vi "Vagus Controller FUZZY ECG Continuous Keithley.vi"() -> ()   [LabVIEW 2020]
uses:
  <instrlib>/Keithley 622x LV 2009/Utility/Typedefs/KE622x -- Instrument Type.ctl
  <instrlib>/Keithley 622x LV 2009/Typedefs/KE622x -- On Off Control.ctl
  <instrlib>/Keithley 622x LV 2009/Configure/Output/Typedefs/KE6221 -- Output Response.ctl
  <instrlib>/Keithley 622x LV 2009/Configure/Source/Typedefs/KE622x -- Current Range.ctl
  <instrlib>/Keithley 622x LV 2009/Configure/Source/Typedefs/KE622x -- Current Ranges.ctl
  <instrlib>/Keithley 622x LV 2009/Configure/Source/Typedefs/KE622x -- Voltage Limit.ctl
  <instrlib>/Keithley 622x LV 2009/Utility/Typedefs/KE622x -- Serial Port Settings.ctl
  <instrlib>/Keithley 622x LV 2009/Configure/Source/Typedefs/KE622x -- Current Level.ctl
  <vilib>/Analysis/baseanly.llb/Mean (DBL).vi
  <vilib>/measure/mascope.llb/Pulse Measurements 1 chan.vi
  <vilib>/addons/Fuzzy Logic/FL Fuzzy Controller (MISO).vi
  <vilib>/Utility/file.llb/Write Delimited Spreadsheet (DBL).vi
  <vilib>/measure/NI_MAPro.lvlib
  <vilib>/addons/Fuzzy Logic/NI_Fuzzy_Logic_API.lvlib
  <instrlib>/Keithley 622x LV 2009/Keithley 622x.lvlib
  <vilib>/Analysis/NI_AALBase.lvlib
panel:
  out "Charge\nDelivered (mC)":dbl
  in  "Reset Charge":bool
  in  "Num Samples\nHR Median":i64 max=1000
  in  "Num Samples\nDC Remove":i64 max=1000
  in  "File Name":string
  in  "Pulse \nPolarity":u16(ring)=1 items=["low pulse", "high pulse"]
  out "Smoothed HR:":dbl format="%#_4g"
  out "Rules Used by Fuzzy Controller":cluster{"Color Box":u32, string}[](array[cluster])
  in  "Activate Controller":bool
  in  "Gain Multiplier":ext
  in  "HR Beat\nThreshold (V)":dbl
  out "?":bool
  out "Measured HR :":dbl format="%#_4g"
  out "HR Waveform":waveform(dbl)(graph)
  in  "Min Current (mA)":dbl
  in  "Max Current (mA)":dbl
  in  "Length of \nBuffer (s)":dbl
  out "Block Output (mA)":ext(graph)
  out "HR Chart":cluster{dbl, "HR Setpoint":i64}(graph)
  in  "HR Setpoint":i64(slide)=200 min=100 max=450 step=1 scale=175.0..375.0
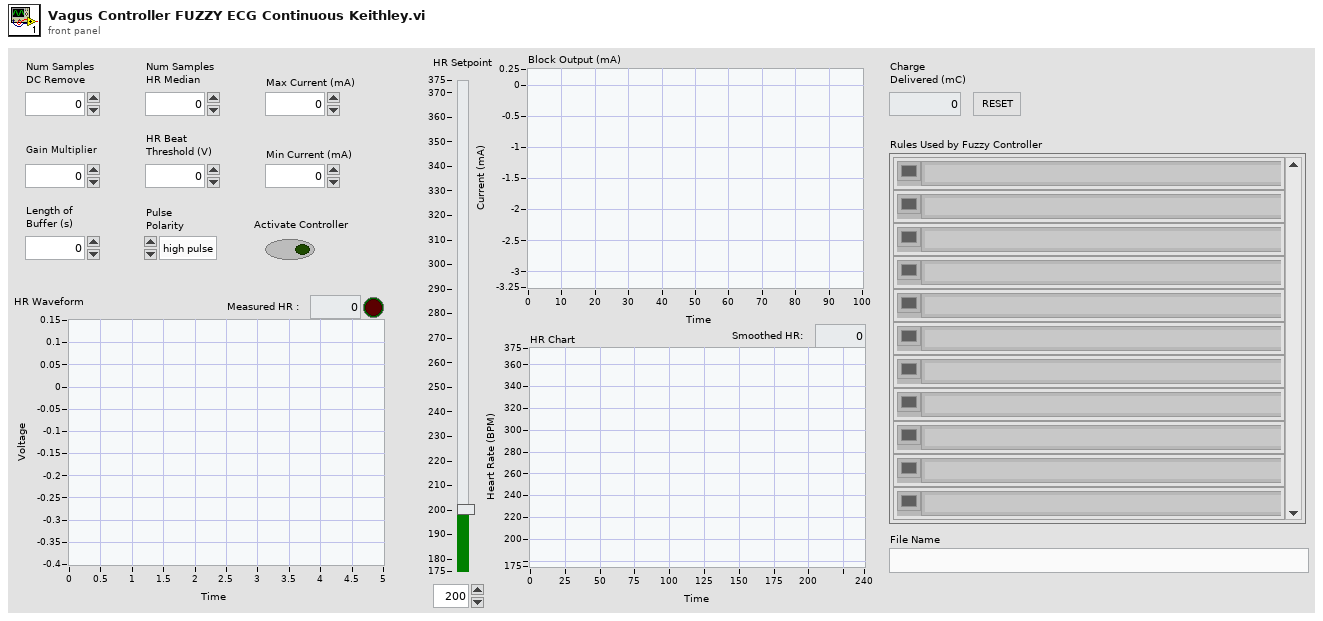
[diagram p1: front panel]
types:
  T1 = typedef "Keithley 622x.lvlib/KE622x -- Current Level.ctl" = dbl
  T2 = typedef "Keithley 622x.lvlib/KE622x -- On Off Control.ctl" = enum16{"Off", "On"}
  T3 = typedef "Keithley 622x.lvlib/KE622x -- Serial Port Settings.ctl" = cluster{"Read Term Char":enum16{"CR", "LF", "CR + LF", "LF + CR"}, "Baud Rate":enum16{"300", "600", "1200", "2400", "4800", "9600", "19200", "38400", "57600", "115200"}, "Flow Control\n(XON / XOFF)":enum16{"Off", "On"}}
  T4 = typedef "Keithley 622x.lvlib/KE622x -- Voltage Limit.ctl" = dbl
  T5 = typedef "Keithley 622x.lvlib/KE622x -- Current Range.ctl" = cluster{"Auto Range?":bool, "Man / Selected\nRange":T6}
  T6 = typedef "Keithley 622x.lvlib/KE622x -- Current Ranges.ctl" = enum16{"2nA", "20nA", "200nA", "2uA", "20uA", "200uA", "2mA", "20mA", "100mA"}
  T7 = typedef "Keithley 622x.lvlib/KE6221 -- Output Response.ctl" = enum16{"Fast", "Slow"}
  T8 = typedef "Keithley 622x.lvlib/KE622x -- Instrument Type.ctl" = enum16{"KE6220", "KE6221"}
  T9 = enum16{"open", "replace", "create", "open or create", "replace or create", "replace or create with confirmation"}
  T10 = typedef "NI_Fuzzy_Logic_API.lvlib/FL System.ctl" = cluster{"input variables":T11[], "output variables":T11[], "rules":T14[], "defuzzification method":T20, "description":string, "user MF interpolating polynomials":T21[]}
  T11 = typedef "NI_Fuzzy_Logic_API.lvlib/FL Variable.ctl" = cluster{"name":string, "range":dbl[], "MFs":T12[]}
  T12 = typedef "NI_Fuzzy_Logic_API.lvlib/FL Membership Function.ctl" = cluster{"name":string, "shape":T13, "points":dbl[], "color":u32, "user-defined shape index":i32}
  T13 = typedef "NI_Fuzzy_Logic_API.lvlib/FL Membership Function Shape.ctl" = u16
  T14 = typedef "NI_Fuzzy_Logic_API.lvlib/FL Rule.ctl" = cluster{"antecedents":T15[], "antecedent connective":T17, "consequents":T18[], "consequent implication":T19, "degree of support":dbl}
  T15 = typedef "NI_Fuzzy_Logic_API.lvlib/FL Antecedent.ctl" = cluster{"Var Index":i32, "MF Index":i32, "Cond":T16}
  T16 = typedef "NI_Fuzzy_Logic_API.lvlib/FL Modifier.ctl" = u16
  T17 = typedef "NI_Fuzzy_Logic_API.lvlib/FL Antecedent Connective.ctl" = u16
  T18 = typedef "NI_Fuzzy_Logic_API.lvlib/FL Consequent.ctl" = cluster{"Var Index":i32, "MF Index":i32, "Cond":T16}
  T19 = typedef "NI_Fuzzy_Logic_API.lvlib/FL Consequent Implication.ctl" = u16
  T20 = typedef "NI_Fuzzy_Logic_API.lvlib/FL Defuzzification.ctl" = u16
  T21 = typedef "NI_Fuzzy_Logic_API.lvlib/FL Interpolating polynomials.ctl" = cluster{"X":dbl[], "Y":dbl[], "Y(x) coeff":dbl[][], "X(y) coeff":dbl[][], "Area(y) coeff":dbl[][], "coa_x(y) coeff":dbl[][]}
  T22 = cluster{"HR Beat\nThreshold (V)":dbl, "HR Beat\nThreshold (V)":dbl, "HR Beat\nThreshold (V)":dbl, "ref units":u16}
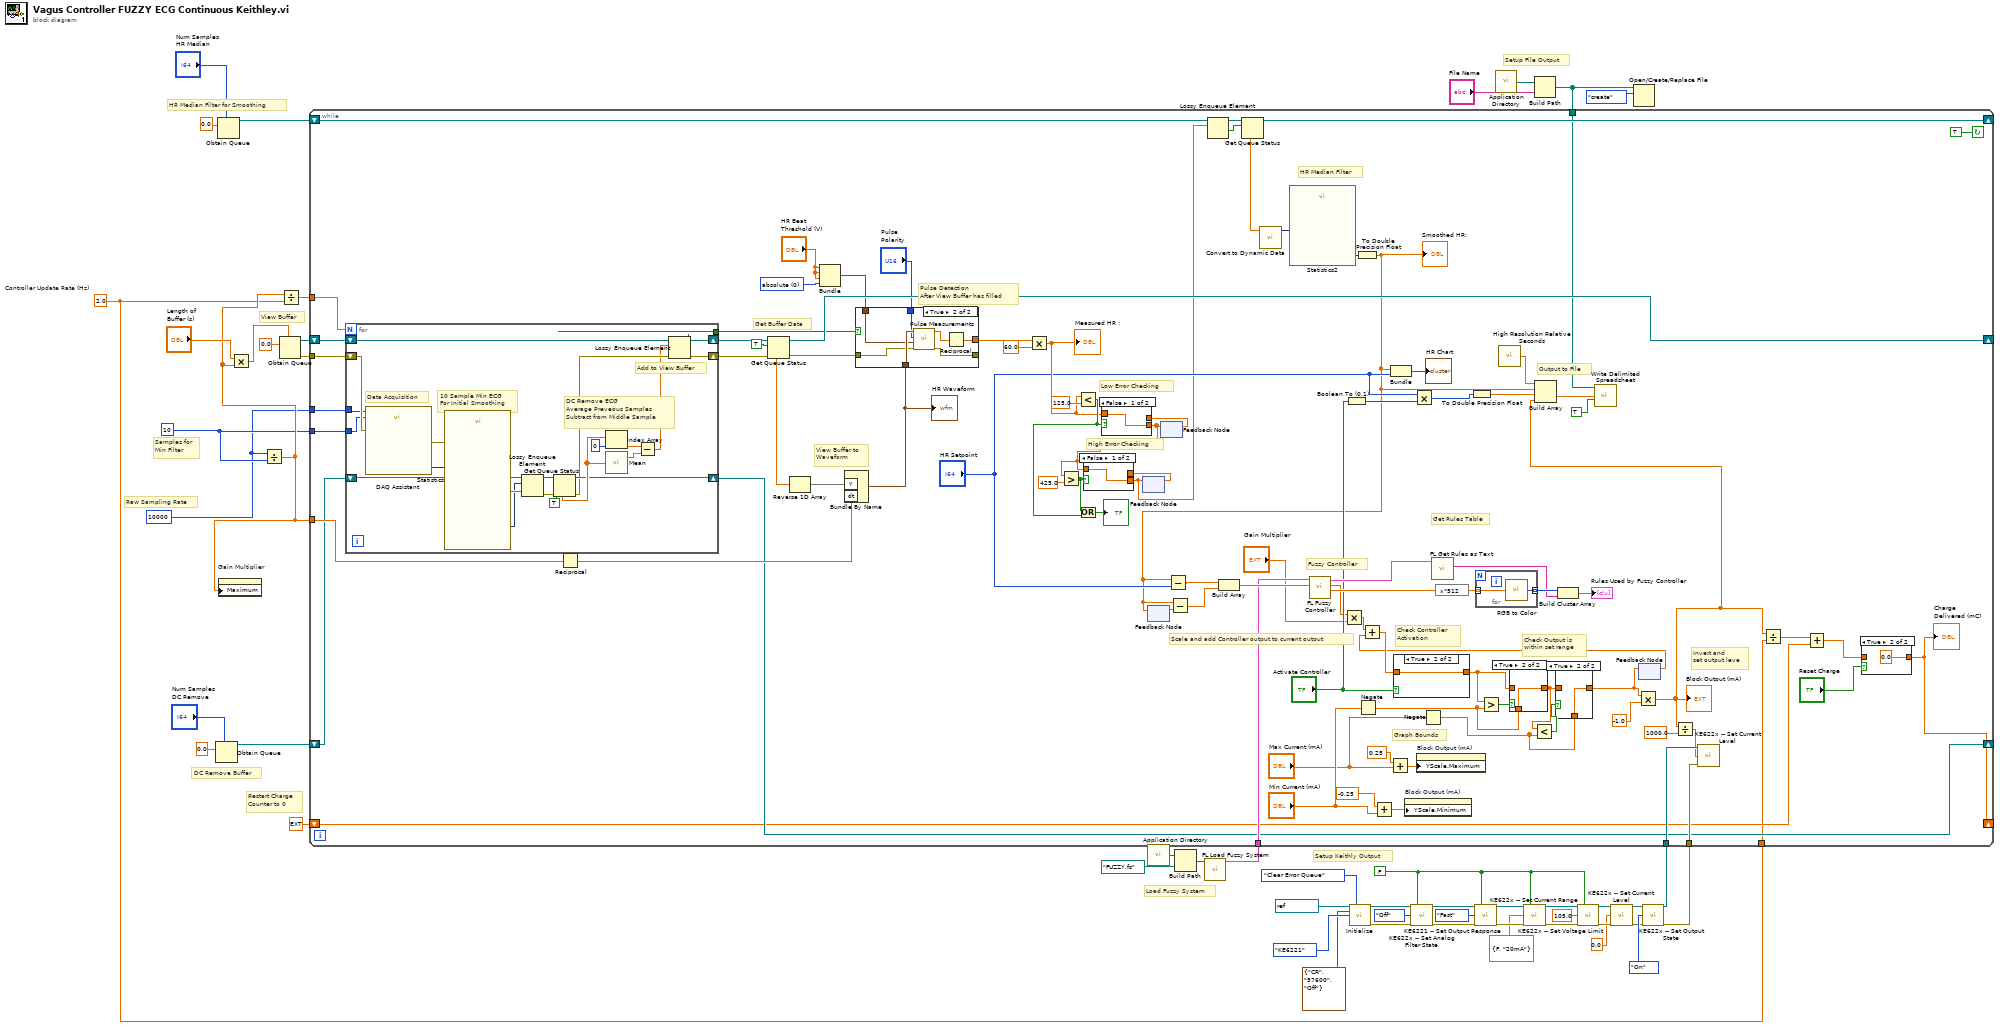
[diagram p0: block diagram]
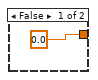
[diagram p7: hidden frame]
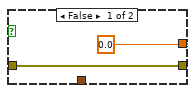
[diagram p8: hidden frame]
diagram:
  w2 = 2.0  # Controller Update Rate (Hz)
  w7 = i64 10000 ("x")
  w8 = i64 10 ("y")
  w24 = FALSE ("Check For SCPI Errors? (T)")
  # "Restart Charge\nCounter to 0"
  # "Setup Keithly Output"
  # "Load Fuzzy System"
  # "Setup File Output"
  # "DC Remove Buffer"
  # "View Buffer"
  # "Raw Sampling Rate"
  # "Samples for\nMin Filter"
  # "HR Median Filter for Smoothing"
  n1 = Obtain Queue(max queue size (-1, unlimited)="Num Samples\nDC Remove", element data type=0.0 ("x")) -> (queue out=w4:refnum<queue>)  [unwired: 3 in, 2 out]
  n2 = Obtain Queue(max queue size (-1, unlimited)="Num Samples\nHR Median", element data type=0.0 ("x")) -> (queue out=w42:refnum<queue>)  [unwired: 3 in, 2 out]
  n3 = Divide(x=w7, y=w8) -> (x/y=w45:dbl)
  n4 = property on="Gain Multiplier" class="DigNum (strict)"("Maximum"=w45) -> ()  [unwired: 2 in, 2 out]
  n5 = Multiply(x="Length of \nBuffer (s)", y=w45) -> (x*y=w47:dbl)
  n6 = Obtain Queue(max queue size (-1, unlimited)=w47, element data type=0.0 ("x")) -> (queue out=w50:refnum<queue>, error out=w49:errorcluster)  [unwired: 3 in, 1 out]
  n7 = Divide(x=w45, y=w2) -> (x/y=w44:dbl)
  n8 = call <vilib>:"Application Directory.vi"() -> ("Application Directory"=w11:path)
  n9 = Build Path(base path=w11, name or relative path=path "FUZZY.fs" ("file path")) -> (appended path=w10:path)
  n10 = call <vilib>:"FL Load Fuzzy System.vi"("file path"=w10) -> ("fuzzy system out"=w41:T10)  [unwired: 9 in, 1 out]
  n11 = call <instrlib>:"Initialize.vi"("VISA resource name"=refnum<visa-resource-name> "COM4", "Error Queue Option"=enum16{"Clear Error Queue", "Error Query"}."Clear Error Queue", "RS-232 Settings"=T3 {"Read Term Char"=enum."CR", "Baud Rate"=enum."57600", "Flow Control\n(XON / XOFF)"=enum."Off"}, "Instrument Type"=KE622x_--_Instrument_Type."KE6221") -> ("VISA resource name out"=w35:refnum<visa-resource-name>, "error out"=w34:errorcluster)  [unwired: 10 in]
  n12 = call <instrlib>:"KE622x -- Set Analog Filter State.vi"("Resource In"=w35, "Check For SCPI Errors? (T)"=w24, "Analog Filter State"=KE622x_--_On_Off_Control."Off", "error in (no error)"=w34) -> ("Resource Out (dupl)"=w33:refnum<visa-resource-name>, "error out"=w32:errorcluster)  [unwired: 10 in]
  n13 = call <instrlib>:"KE6221 -- Set Output Response.vi"("Resource In"=w33, "Check For SCPI Errors? (T)"=w24, "KE6221 Output Response"=KE6221_--_Output_Response."Fast", "error in (no error)"=w32) -> ("Resource Out (dupl)"=w27:refnum<visa-resource-name>, "error out"=w26:errorcluster)  [unwired: 10 in]
  n14 = call <vilib>:"Application Directory.vi"() -> ("Application Directory"=w37:path)
  n15 = call <instrlib>:"KE622x -- Set Current Range.vi"("Resource In"=w27, "Check For SCPI Errors? (T)"=w24, "Current Range In"=T5 {"Auto Range?"=FALSE, "Man / Selected\nRange"=enum."20mA"}, "error in (no error)"=w26) -> ("Resource Out (dupl)"=w23:refnum<visa-resource-name>, "error out"=w22:errorcluster)  [unwired: 9 in, 1 out]
  n16 = Build Path(base path=w37, name or relative path="File Name") -> (appended path=w40:path)
  n17 = call <instrlib>:"KE622x -- Set Voltage Limit.vi"("Resource In"=w23, "Check For SCPI Errors? (T)"=w24, "Voltage Limit (V)"=T4 105.0, "error in (no error)"=w22) -> ("Resource Out (dupl)"=w15:refnum<visa-resource-name>, "error out"=w14:errorcluster)  [unwired: 10 in]
  n18 = call <instrlib>:"KE622x -- Set Current Level.vi"("Resource In"=w15, "Current Level (A) In"=T1 0.0, "error in (no error)"=w14) -> ("Resource Out (dupl)"=w16:refnum<visa-resource-name>, "error out"=w13:errorcluster)  [unwired: 10 in, 1 out]
  n19 = Open/Create/Replace File(file path (use dialog)=w40, operation (0:open)=T9."create") -> ()  [unwired: 4 in, 3 out]
  n20 = call <instrlib>:"KE622x -- Set Output State.vi"("Resource In"=w16, "Output State"=KE622x_--_On_Off_Control."On", "error in (no error)"=w13) -> ("Resource Out (dupl)"=w18:refnum<visa-resource-name>, "error out"=w17:errorcluster)  [unwired: 11 in]
  n21 = while {
    shift-right: [w138] -> _
    shift-left: w50 -> [w141]
    tunnel: w45 -> [w110]
    tunnel: w44 -> [w128]
    tunnel: w8 -> [w113]
    tunnel: w7 -> [w112]
    shift-right: [w92] -> _
    shift-left: w42 -> [w91]
    tunnel: w41 -> [w86]
    tunnel: w40 -> [w85]
    tunnel: w18 -> [w79]
    tunnel: w17 -> [w78]
    shift-right: [w73] -> _
    shift-left: w4 -> [w74]
    shift-right: [w56] -> _
    shift-left: ext 0.0 -> [w59]
    tunnel: w2 -> [w54]
    tunnel: w49 -> [w134]
    stop <- TRUE continue-if-true
    w131 = u16 0 items=["absolute", "percent"] ("ref units")
    # "Get Buffer Data"
    # "Graph Bounds"
    # "Invert and\nset output leve"
    # "Check Output is \nwithin set range"
    # "Scale and add Controller output to current output"
    # "Check Controller\nActivation"
    # "Get Rules Table"
    # "Fuzzy Controller"
    # "Output to File"
    # "High Error Checking"
    # "Low Error Checking"
    # "HR Median Filter"
    # "View Buffer to\nWaveform"
    # "Pulse Detection\nAfter View Buffer has filled"
    n22 = for {
      N: w128 -> [_]
      tunnel: [w177] -> w132
      shift-right: [w179] -> w140
      shift-left: w141 -> [w180]
      shift-right: [w178] -> w139
      shift-left: w134 -> [w176]
      tunnel: w113 -> [w173]
      tunnel: w112 -> [w172]
      shift-right: [w164] -> w73
      shift-left: w74 -> [w165]
      # "Add to View Buffer"
      # "DC Remove ECG\nAverage Preveous Samples\nSubtract from Middle Sample"
      # "10 Sample Min ECG\nFor Initial Smoothing"
      # "Data Acquisition"
      n23 = call "DAQ Assistant"("rate"=w172, "number of samples"=w173, "error in"=w176) -> ("data"=w174:dynamicdata, "error out"=w175:errorcluster)  [unwired: 13 in, 2 out]
      n24 = call "Statistics"("Signals"=w174, "error in (no error)"=w175) -> ("Median"=w159:dynamicdata, "error out"=w163:errorcluster)  [unwired: 20 in, 4 out]
      n25 = Lossy Enqueue Element(queue=w165, element=w159, error in (no error)=w163) -> (queue out=w171:refnum<queue>, error out=w170:errorcluster)  [unwired: 2 out]
      n26 = Get Queue Status(queue=w171, return elements? (F)=TRUE, error in (no error)=w170) -> (queue out=w164:refnum<queue>, error out=w162:errorcluster, elements=w168:dbl[])  [unwired: 5 out]
      n27 = Index Array(array=w168, index=0) -> (element=w167:dbl)
      n28 = call-poly <vilib>:"Mean.vi"("X"=w168) -> ("mean"=w166:dbl)  [unwired: 1 out]
      n29 = Subtract(x=w167, y=w166) -> (x-y=w161:dbl)
      n30 = Lossy Enqueue Element(queue=w180, element=w161, error in (no error)=w162) -> (queue out=w179:refnum<queue>, overflow?=w177:bool, error out=w178:errorcluster)  [unwired: 1 out]
    }
    n31 = Reciprocal(x=w110) -> (1/x=w111:dbl)
    n32 = Get Queue Status(queue=w140, return elements? (F)=TRUE, error in (no error)=w139) -> (queue out=w138:refnum<queue>, error out=w133:errorcluster, elements=w52:dbl[])  [unwired: 5 out]
    n33 = Reverse 1D Array(array=w52) -> (reversed array=w51:dbl[])
    n34 = Bundle("HR Beat\nThreshold (V)"="HR Beat\nThreshold (V)", "HR Beat\nThreshold (V)"="HR Beat\nThreshold (V)", "HR Beat\nThreshold (V)"="HR Beat\nThreshold (V)", "ref units"=w131) -> (w130:T22)  [unwired: 1 out]
    n35 = Bundle By Name("Y"=w51, "dt"=w111) -> (w135:waveform(dbl))  [unwired: 1 in]
    "HR Waveform" <- w135
    n36 = case shown="True" w132 {
      tunnel: w135 -> [_ w189]
      tunnel: [0.0 ("amplitude") w187] -> w129
      tunnel: w133 -> [w181 w186]
      tunnel: w130 -> [_ w185]
      tunnel: "Pulse \nPolarity" -> [_ w184]
      tunnel: [w181 w183] -> _
      frame False {
      }
      frame True {
        n37 = call-poly <vilib>:"Pulse Measurements.vi"("error in (no error)"=w186, "reference levels"=w185, "polarity (high)"=w184, "signal in"=w189) -> ("error out"=w183:errorcluster, "period"=w188:dbl)  [unwired: 3 in, 3 out]
        n38 = Reciprocal(x=w188) -> (1/x=w187:dbl)
      }
    }
    n39 = Multiply(x=w129, y=60.0 ("x")) -> (x*y=w103:dbl)
    "Measured HR :" <- w103
    n40 = Less?(x=w103, y=125.0) -> (x < y?=w105:bool)
    n41 = feedback #1() -> (w93:dbl)  [unwired: 1 in]
    n42 = feedback #2() -> (w101:dbl)  [unwired: 1 in]
    n43 = feedback #3() -> (w102:dbl)  [unwired: 1 in]
    n44 = case shown="False" w105 {
      tunnel: w103 -> [w149 _]
      tunnel: [w149 w150] -> w108
      tunnel: w102 -> [_ w150]
      frame False {
      }
      frame True {
      }
    }
    n45 = Greater?(x=w108, y=425.0) -> (0:w106:bool)
    n46 = Or(x=w106, y=w105) -> (x .or. y?=→"?":bool)
    n47 = case shown="False" w106 {
      tunnel: w108 -> [w147 _]
      tunnel: [w147 w148] -> w72
      tunnel: w93 -> [_ w148]
      frame False {
      }
      frame True {
      }
    }
    n48 = feedback-in #1(w72) -> ()
    n49 = feedback-in #3(w108) -> ()
    n50 = Lossy Enqueue Element(queue=w91, element=w72) -> (queue out=w97:refnum<queue>, overflow?=w96:bool)  [unwired: 1 in, 2 out]
    n51 = Get Queue Status(queue=w97, return elements? (F)=w96) -> (queue out=w92:refnum<queue>, elements=w95:dbl[])  [unwired: 1 in, 6 out]
    n52 = call "Convert to Dynamic Data"("Array"=w95) -> ("Dynamic Data Type"=w94:dynamicdata)  [unwired: 3 in]
    n53 = call "Statistics2"("Signals"=w94) -> ("Median"=w75:dynamicdata)  [unwired: 24 in, 2 out]
    n54 = Boolean To (0,1)(Boolean="Activate Controller") -> (0, 1=w80:i16)
    n55 = To Double Precision Float(number=w75) -> (double precision float=w71:dbl)
    "Smoothed HR:" <- w71
    n56 = feedback-in #2(w71) -> ()
    n57 = Subtract(x=w71, y="HR Setpoint") -> (x-y=w99:dbl)
    n58 = Subtract(x=w71, y=w101) -> (x-y=w98:dbl)
    n59 = Build Array(w99, w98) -> (w100:dbl[])
    n60 = call-poly <vilib>:"FL Fuzzy Controller.vi"("input values"=w100, "fuzzy system in"=w86) -> ("rule weights"=w122:dbl[], "output value"=w69:dbl, "fuzzy system out"=w126:T10)  [unwired: 5 in, 2 out]
    n61 = Multiply(x=w69, y="Gain Multiplier") -> (x*y=w68:ext)
    n62 = Negate(x="Min Current (mA)") -> (-x=w65:dbl)
    n63 = Add(x=-0.25 ("y"), y="Min Current (mA)") -> (x+y=w62:dbl)
    n64 = Add(x=0.25, y="Max Current (mA)") -> (x+y=w61:dbl)
    n65 = Bundle "Bundle"(w71, "HR Setpoint"="HR Setpoint") -> (→"HR Chart":cluster{dbl, "HR Setpoint":i64})  [unwired: 1 out]
    n66 = property on="Block Output (mA)" class="WFChart (strict)"("YScale.Minimum"=w62) -> ()  [unwired: 2 in, 2 out]
    n67 = Multiply(x="HR Setpoint", y=w80) -> (x*y=w81:i64)
    n68 = property on="Block Output (mA)" class="WFChart (strict)"("YScale.Maximum"=w61) -> ()  [unwired: 2 in, 2 out]
    n69 = Negate(x="Max Current (mA)") -> (-x=w63:dbl)
    n70 = call <vilib>:"FL Get Rules as Text.vi"("fuzzy system in"=w126) -> ("rules as text"=w121:string[])  [unwired: 8 in, 2 out]
    n71 = expression code="x*512"(w122) -> (w125:dbl[])
    n72 = To Double Precision Float(number=w81) -> (double precision float=w88:dbl)
    n73 = for {
      tunnel: w125 -> [w155] mode=indexing
      tunnel: [w156] -> w124 mode=indexing
      n74 = call <vilib>:"RGB to Color.vi"("G"=w155) -> ("Color"=w156:u32)  [unwired: 2 in]
    }
    n75 = call <vilib>:"High Resolution Relative Seconds.vi"() -> ("relative seconds"=w84:dbl)
    n76 = Build Cluster Array(w124, w121) -> (→"Rules Used by Fuzzy Controller":cluster{"Color":u32, string}[])
    n77 = feedback #4() -> (w120:ext)  [unwired: 1 in]
    n78 = Add(x=w68, y=w120) -> (x+y=w127:ext)
    n79 = case shown="True" "Activate Controller" {
      tunnel: w127 -> [_ w158]
      tunnel: [0.0 ("output variable") w158] -> w116
      frame False {
      }
      frame True {
      }
    }
    n80 = Greater?(x=w116, y=w65) -> (0:w119:bool)
    n81 = case shown="True" w119 {
      tunnel: w116 -> [w153 _]
      tunnel: [w153 w154] -> w117
      tunnel: w65 -> [_ w154]
      frame False {
      }
      frame True {
      }
    }
    n82 = Less?(x=w117, y=w63) -> (x < y?=w118:bool)
    n83 = case shown="True" w118 {
      tunnel: w117 -> [w151 _]
      tunnel: [w151 w152] -> w114
      tunnel: w63 -> [_ w152]
      frame False {
      }
      frame True {
      }
    }
    n84 = Multiply(x=w114, y=-1.0) -> (x*y=w53:ext)
    "Block Output (mA)" <- w53
    n85 = Build Array(w84, w71, w88, w53) -> (w89:ext[])
    n86 = call-poly <vilib>:"Write Delimited Spreadsheet.vi"("file path (dialog if empty)"=w85, "1D data"=w89, "append to file? (new file:F)"=TRUE) -> ()  [unwired: 11 in, 2 out]
    n87 = feedback-in #4(w114) -> ()
    n88 = Divide(x=w53, y=1000.0) -> (x/y=w60:ext)
    n89 = call <instrlib>:"KE622x -- Set Current Level.vi"("Resource In"=w79, "Current Level (A) In"=w60, "error in (no error)"=w78) -> ()  [unwired: 10 in, 3 out]
    n90 = Divide(x=w53, y=w54) -> (x/y=w58:ext)
    n91 = Add(x=w58, y=w59) -> (x+y=w57:ext)
    n92 = case shown="True" "Reset Charge" {
      tunnel: w57 -> [w145 _]
      tunnel: [w145 0.0] -> w56
      frame False {
      }
      frame True {
      }
    }
    "Charge\nDelivered (mC)" <- w56
  }
